vi "Get Provided Interface and Service Class.vi"(8 "error in (no error)":errorcluster, 11 "instrument in":refnum<class "Fake Instrument.lvclass">) -> (0 "error out":errorcluster, 1 "service class":string, 2 "provided interface":string, 3 "instrument out":refnum<class "Fake Instrument.lvclass">)   [LabVIEW 2020, in "MeasurementServerTests.lvlib" / "Fake Instrument.lvclass"]
uses:
  Fake Instrument.lvclass
  Fake Instrument.lvclass/Fake Instrument.ctl
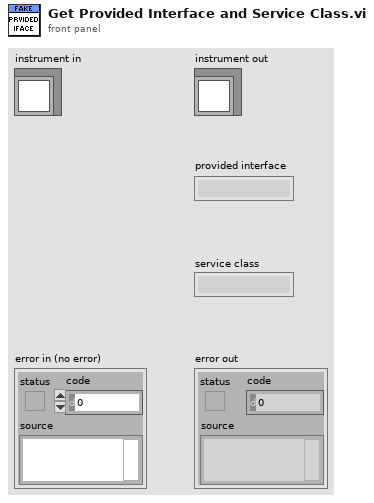
[diagram p1: front panel]
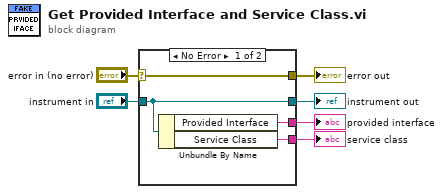
[diagram p0: block diagram]
diagram:
  n1 = case shown="No Error" "error in (no error)" {
    selector: "error in (no error)" -> [w10 w11]
    tunnel: "instrument in" -> [w9 w12]
    tunnel: [w9 w12] -> w5
    tunnel: [w10 w11] -> w3
    tunnel: [w8 _] -> w2
    tunnel: [w7 _] -> w1
    frame No Error {
      n2 = Unbundle By Name(w9) -> ("Provided Interface"=w8:string, "Service Class"=w7:string)
    }
    frame Error {
    }
  }
  "error out" <- w3
  "instrument out" <- w5
  "provided interface" <- w2
  "service class" <- w1
